vi "sub_getComputerMove.vi"(4 "computer symbol":string, 6 "player symbol":string, 11 "control references (in)":refnum<vi>[](array[refnum])) -> (2 "computer move":i32, 3 "control references (out)":refnum<vi>[](array[refnum]))   [LabVIEW 2018]
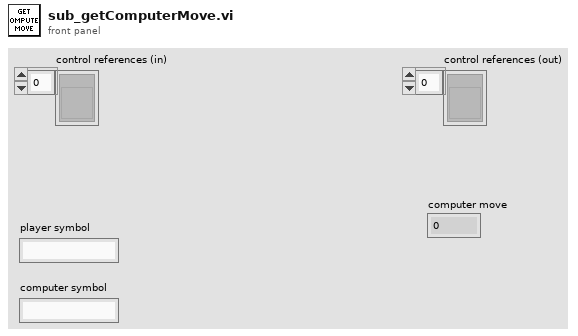
[diagram p1: front panel]
types:
  T1 = cluster{"corner indexes":i32[], "side indexes":i32[], "center index":i32}
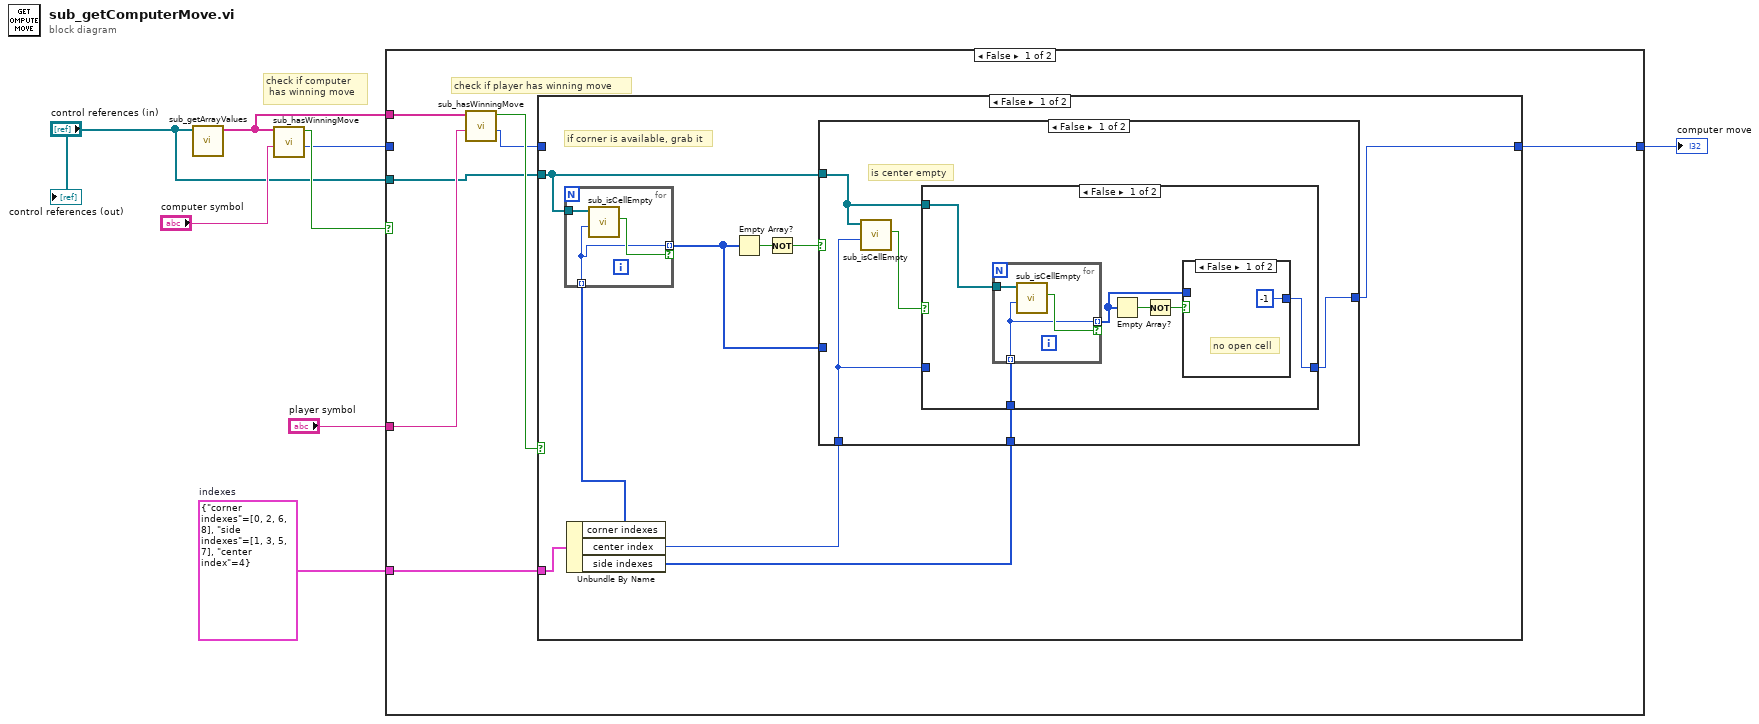
[diagram p0: block diagram]
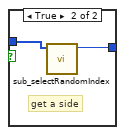
[diagram p2: hidden frame]
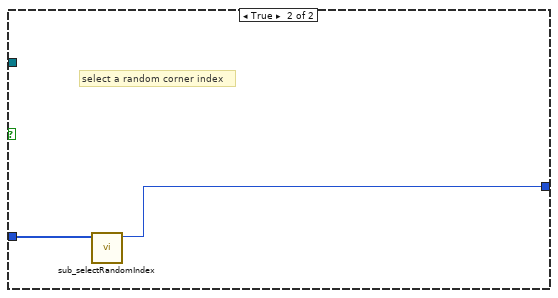
[diagram p4: hidden frame]
diagram:
  w4 = T1 {"corner indexes"=[0, 2, 6, 8], "side indexes"=[1, 3, 5, 7], "center index"=4}  # indexes
  # "check if computer\n has winning move"
  n1 = call "sub_getArrayValues.vi"("controls"="control references (in)") -> ("array"=w6:string[])  [unwired: 10 in]
  n2 = call "sub_hasWinningMove.vi"("player"="computer symbol", "array"=w6) -> ("winning move"=w1:i32, "has winning move"=w7:bool)  [unwired: 8 in]
  n3 = case shown="False" w7 {
    tunnel: w6 -> [w15 _]
    tunnel: "player symbol" -> [w14 _]
    tunnel: w4 -> [w12 _]
    tunnel: "control references (in)" -> [w11 _]
    tunnel: [w10 w49] -> w2
    tunnel: w1 -> [_ w49]
    frame False {
      # "check if player has winning move"
      n4 = call "sub_hasWinningMove.vi"("player"=w14, "array"=w15) -> ("winning move"=w9:i32, "has winning move"=w13:bool)  [unwired: 8 in]
      n5 = case shown="False" w13 {
        tunnel: w12 -> [w24 _]
        tunnel: w11 -> [w20 _]
        tunnel: [w22 w48] -> w10
        tunnel: w9 -> [_ w48]
        frame False {
          # "if corner is available, grab it"
          n6 = Unbundle By Name(w24) -> ("corner indexes"=w23:i32[], "center index"=w21:i32, "side indexes"=w16:i32[])
          n7 = for {
            tunnel: w20 -> [w47]
            tunnel: w23 -> [w45] mode=indexing
            tunnel: [w45] -> w17 mode=indexing if=w46
            n8 = call "sub_isCellEmpty.vi"("selection index"=w45, "control references"=w47) -> ("empty?"=w46:bool)  [unwired: 9 in]
          }
          n9 = Empty Array?(array=w17) -> (empty?=w19:bool)
          n10 = Not(x=w19) -> (.not. x?=w18:bool)
          n11 = case shown="False" w18 {
            tunnel: [w27 w43] -> w22
            tunnel: w21 -> [w28 _]
            tunnel: w20 -> [w26 _]
            tunnel: w17 -> [_ w44]
            tunnel: w16 -> [w25 _]
            frame False {
              # "is center empty"
              n12 = call "sub_isCellEmpty.vi"("selection index"=w28, "control references"=w26) -> ("empty?"=w29:bool)  [unwired: 9 in]
              n13 = case shown="False" w29 {
                tunnel: w28 -> [_ w42]
                tunnel: [w30 w42] -> w27
                tunnel: w26 -> [w35 _]
                tunnel: w25 -> [w34 _]
                frame False {
                  n14 = for {
                    tunnel: [w39] -> w31 mode=indexing if=w41
                    tunnel: w35 -> [w40]
                    tunnel: w34 -> [w39] mode=indexing
                    n15 = call "sub_isCellEmpty.vi"("selection index"=w39, "control references"=w40) -> ("empty?"=w41:bool)  [unwired: 9 in]
                  }
                  n16 = Empty Array?(array=w31) -> (empty?=w33:bool)
                  n17 = Not(x=w33) -> (.not. x?=w32:bool)
                  n18 = case shown="False" w32 {
                    tunnel: w31 -> [_ w38]
                    tunnel: [-1 ("random selected index") w37] -> w30
                    frame False {
                      # "no open cell"
                    }
                    frame True {
                      # "get a side"
                      n19 = call "sub_selectRandomIndex.vi"("indexes"=w38) -> ("random selected index"=w37:i32)  [unwired: 10 in]
                    }
                  }
                }
                frame True {
                }
              }
            }
            frame True {
              # "select a random corner index"
              n20 = call "sub_selectRandomIndex.vi"("indexes"=w44) -> ("random selected index"=w43:i32)  [unwired: 10 in]
            }
          }
        }
        frame True {
        }
      }
    }
    frame True {
    }
  }
  "computer move" <- w2
  "control references (out)" <- "control references (in)"
